vi "Jenkins - Run Script.vi"(8 "error in (no error)":errorcluster, 9 "Parameters":variant, 10 "Script Job Name (Within Build Script Folder)":string, 11 "IP Address":string) -> (0 "error out":errorcluster, 3 "Text":string)   [LabVIEW 2014]
uses:
  <vilib>/Utility/error.llb/Error Cluster From Error Code.vi
  <vilib>/ErrorRing/Error Ring.xnode
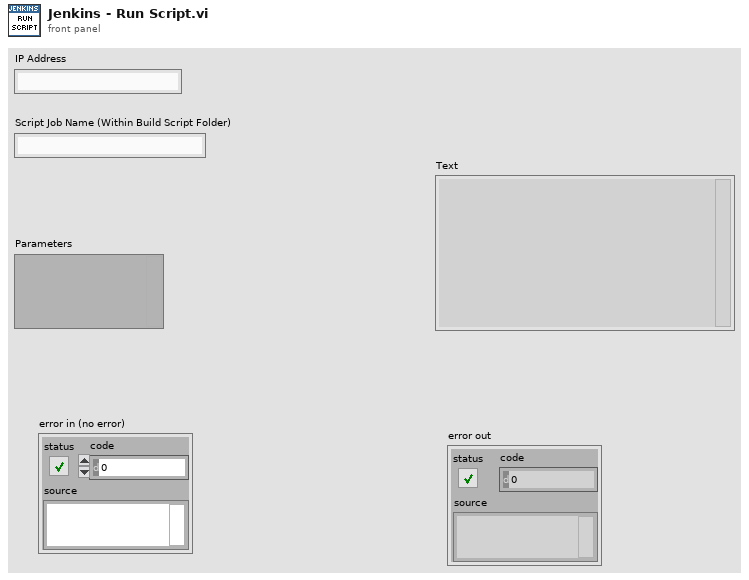
[diagram p1: front panel]
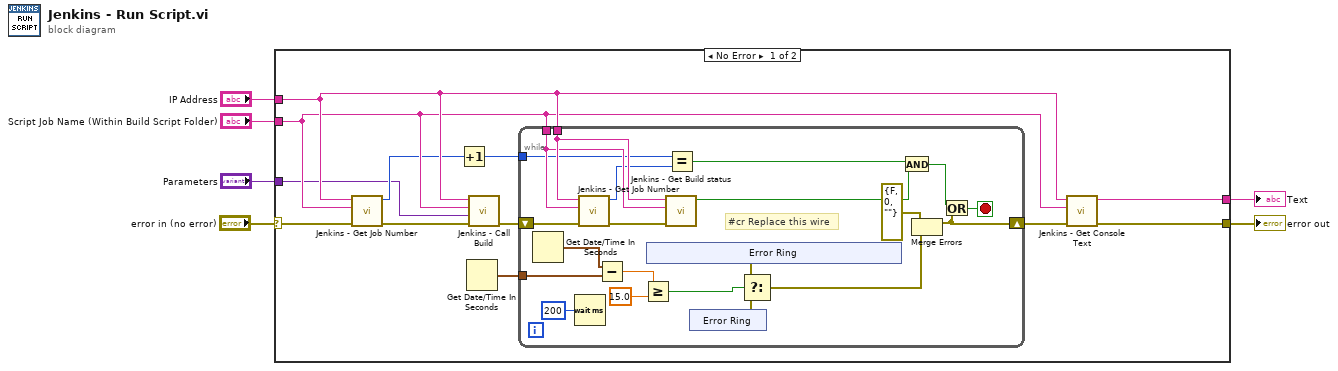
[diagram p0: block diagram]
diagram:
  n1 = case shown="No Error" "error in (no error)" {
    selector: "error in (no error)" -> [w13 w46]
    tunnel: "IP Address" -> [w18 _]
    tunnel: "Script Job Name (Within Build Script Folder)" -> [w16 _]
    tunnel: "Parameters" -> [w10 _]
    tunnel: [w7 w46] -> w3
    tunnel: [w9 _] -> w2
    frame No Error {
      n2 = call "Jenkins - Get Job Number.vi"("error in (no error)"=w13, "Script Job Name (Within Build Script Folder)"=w16, "IP Address"=w18) -> ("error out"=w17:errorcluster, "Job Number"=w12:i32)  [unwired: 7 in]
      n3 = Increment(x=w12) -> (x+1=w11:i32)
      n4 = Get Date/Time In Seconds() -> (seconds since 1Jan1904=w8:timestamp)
      n5 = call "Jenkins - Call Build.vi"("error in (no error)"=w17, "Parameters"=w10, "Script Job Name (Within Build Script Folder)"=w16, "IP Address"=w18) -> ("error out"=w15:errorcluster)  [unwired: 7 in]
      n6 = while {
        tunnel: w18 -> [w37]
        tunnel: w16 -> [w36]
        shift-right: [w24] -> w14
        shift-left: w15 -> [w33]
        tunnel: w11 -> [w34]
        tunnel: w8 -> [w27]
        stop <- w38 stop-if-true
        # "#cr Replace this wire"
        n7 = Get Date/Time In Seconds() -> (seconds since 1Jan1904=w28:timestamp)
        n8 = Wait (ms)(milliseconds to wait=u32 200) -> ()  [unwired: 1 out]
        n9 = call "Jenkins - Get Job Number.vi"("error in (no error)"=w33, "Script Job Name (Within Build Script Folder)"=w36, "IP Address"=w37) -> ("error out"=w32:errorcluster, "Job Number"=w35:i32)  [unwired: 7 in]
        n10 = Subtract(x=w28, y=w27) -> (x-y=w25:dbl)
        n11 = Greater Or Equal?(x=w25, y=15.0) -> (x >= y?=w23:bool)
        n12 = xnode "Error Ring"() -> ("error out"=w21:errorcluster)
        n13 = call "Jenkins - Get Build status.vi"("error in (no error)"=w32, "Script Job Name (Within Build Script Folder)"=w36, "IP Address"=w37) -> ("Done?"=w29:bool)  [unwired: 6 in, 2 out]
        n14 = Equal?(x=w34, y=w35) -> (x = y?=w31:bool)
        n15 = xnode "Error Ring"() -> ("error out"=w22:errorcluster)
        n16 = Select(t=w21, s=w23, f=w22) -> (s? t:f=w20:errorcluster)
        n17 = And(x=w31, y=w29) -> (x .and. y?=w30:bool)
        n18 = Merge Errors(errorcluster {"status"=FALSE, "code"=0, "source"=""} ("error in"), w20) -> (w24:errorcluster)
        n19 = Or(x=w30, y=w24) -> (x .or. y?=w38:bool)
      }
      n20 = call "Jenkins - Get Console Text.vi"("error in (no error)"=w14, "Script Job Name (Within Build Script Folder)"=w16, "IP Address"=w18) -> ("error out"=w7:errorcluster, "Text"=w9:string)  [unwired: 7 in]
    }
    frame Error {
    }
  }
  "error out" <- w3
  "Text" <- w2
